vi "HIOKI PW3390 Conf Efficiency.vi"(0 "VISA Resource":refnum<visa-resource-name>, 1 "Set/Query (F: Set)":bool, 5 "Pin (0: P1)":T1(array[ring])=[enum."P1", enum."P1", enum."P1"], 7 "Pout (0: P1)":T1(array[ring])=[enum."P1", enum."P1", enum."P1"], 11 "error in (no error)":errorcluster, 12 "OPC query (T: ON)":bool=TRUE, 13 "Error Out (F: Off)":bool) -> (4 "VISA Resource out":refnum<visa-resource-name>, 6 "Pin out":T1(array[ring])=[enum."P1", enum."P1", enum."P1"], 8 "Pout out":T1(array[ring])=[enum."P1", enum."P1", enum."P1"], 15 "error out":errorcluster)   [LabVIEW 2009]
doc: "Sets and reads the Efficiency/Loss Calculation Formula. \n\nSet/Query\n Set: Send the setting commands for the device.\n Query: Query the setting of the device.\n\nPin\n Sets the Pin items of the Efficiency/Loss Calculation Formula for CH1 - CH3 in array.\n\nPout\n Sets the Pout items of the Efficiency/Loss Calculation Formula for CH1 - CH3 in array.\n\n<B>Note</B>\n P12/P34/P123 cannot be specified when they cannot be selected because of the wiring setting. Pm can only be specified during the implementation of the Motor Analysis Option and when Pm is selectable."
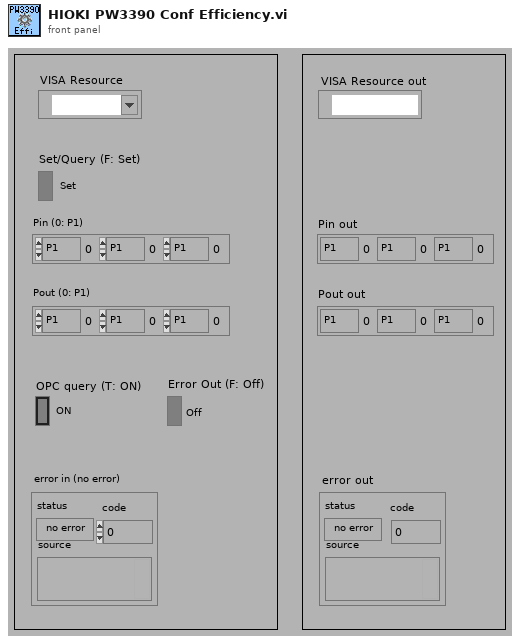
[diagram p1: front panel]
types:
  T1 = enum16{"P1", "P2", "P3", "P4", "P12", "P34", "P123", "Pm"}[]
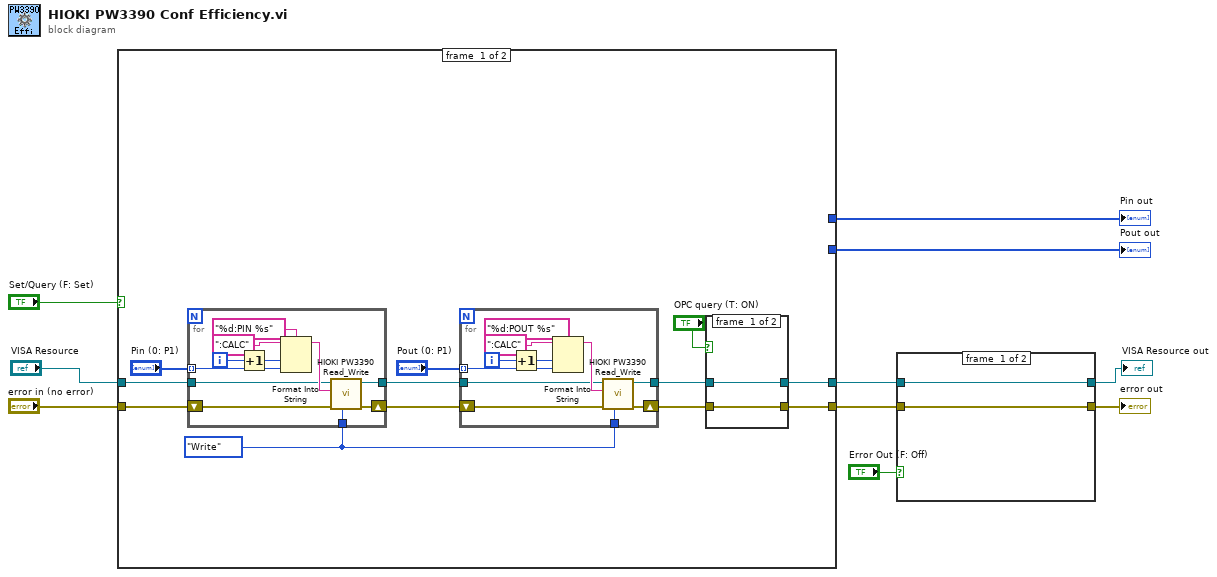
[diagram p0: block diagram]
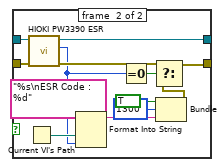
[diagram p2: hidden frame]
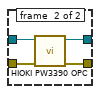
[diagram p3: hidden frame]
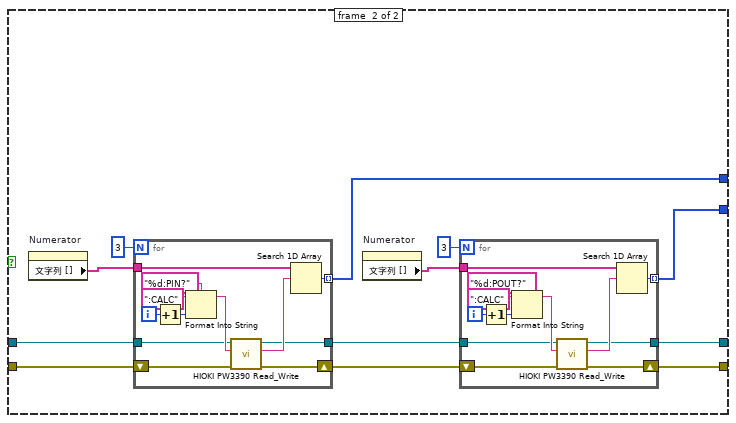
[diagram p4: hidden frame]
diagram:
  n1 = case shown="FALSE" "Set/Query (F: Set)" {
    tunnel: "error in (no error)" -> [w21 w60]
    tunnel: [w11 w53] -> w4
    tunnel: "VISA Resource" -> [w22 w61]
    tunnel: [w12 w57] -> w5
    tunnel: [_ w58] -> w8
    tunnel: [_ w54] -> w7
    frame #0 {
      w18 = enum16{"Read", "Write"}."Write" ("Read/Write")
      n2 = for {
        tunnel: "Pin (0: P1)" -> [w46] mode=indexing
        tunnel: w22 -> [w44]
        shift-right: [w43] -> w20
        shift-left: w21 -> [w42]
        tunnel: [w41] -> w19
        tunnel: w18 -> [w40]
        i -> [w48]
        n3 = Increment(x=w48) -> (x+1=w47:i32)
        n4 = Format Into String(format string="%d:PIN %s", initial string=":CALC", w47, w46) -> (resulting string=w45:string)  [unwired: 1 in, 1 out]
        n5 = call <instrlib>:"HIOKI PW3390 Read_Write.vi"("Read/Write"=w40, "error in (no error)"=w42, "data in"=w45, "VISA Resource"=w44) -> ("error out"=w43:errorcluster, "VISA Resource out"=w41:refnum<visa-resource-name>)  [unwired: 5 in, 1 out]
      }
      n6 = for {
        tunnel: "Pout (0: P1)" -> [w35] mode=indexing
        tunnel: w19 -> [w33]
        shift-right: [w32] -> w13
        shift-left: w20 -> [w31]
        tunnel: [w30] -> w14
        tunnel: w18 -> [w29]
        i -> [w37]
        n7 = Increment(x=w37) -> (x+1=w36:i32)
        n8 = Format Into String(format string="%d:POUT %s", initial string=":CALC", w36, w35) -> (resulting string=w34:string)  [unwired: 1 in, 1 out]
        n9 = call <instrlib>:"HIOKI PW3390 Read_Write.vi"("Read/Write"=w29, "error in (no error)"=w31, "data in"=w34, "VISA Resource"=w33) -> ("error out"=w32:errorcluster, "VISA Resource out"=w30:refnum<visa-resource-name>)  [unwired: 5 in, 1 out]
      }
      n10 = case shown="TRUE" "OPC query (T: ON)" {
        tunnel: [w24 w28] -> w12
        tunnel: [w23 w27] -> w11
        tunnel: w14 -> [w24 w26]
        tunnel: w13 -> [w23 w25]
        frame #0 {
        }
        frame #1 {
          n11 = call <instrlib>:"HIOKI PW3390 OPC.vi"("error in (no error)"=w25, "VISA Resource"=w26) -> ("error out"=w27:errorcluster, "VISA Resource out"=w28:refnum<visa-resource-name>)  [unwired: 7 in, 1 out]
        }
      }
    }
    frame #1 {
      # "Query"
      n12 = property on="Numerator" class="Enum (strict)"() -> ("文字列 []"=w62:string[])  [unwired: 2 in, 2 out]
      n13 = for {
        N: 3 -> [_]
        tunnel: [w86] -> w58 mode=indexing
        tunnel: w62 -> [w84]
        tunnel: w61 -> [w79]
        shift-right: [w77] -> w56
        shift-left: w60 -> [w78]
        tunnel: [w76] -> w59
        i -> [w81]
        n14 = Increment(x=w81) -> (x+1=w75:i32)
        n15 = Format Into String(format string="%d:PIN?", initial string=":CALC", w75) -> (resulting string=w80:string)  [unwired: 1 in, 1 out]
        n16 = call <instrlib>:"HIOKI PW3390 Read_Write.vi"("error in (no error)"=w78, "data in"=w80, "VISA Resource"=w79) -> ("error out"=w77:errorcluster, "data out"=w85:string, "VISA Resource out"=w76:refnum<visa-resource-name>)  [unwired: 6 in]
        n17 = Search 1D Array(1D array=w84, element=w85) -> (index of element=w86:i32)  [unwired: 1 in]
      }
      n18 = property on="Numerator" class="Enum (strict)"() -> ("文字列 []"=w55:string[])  [unwired: 2 in, 2 out]
      n19 = for {
        N: 3 -> [_]
        tunnel: [w74] -> w54 mode=indexing
        tunnel: w55 -> [w72]
        tunnel: w59 -> [w67]
        shift-right: [w65] -> w53
        shift-left: w56 -> [w66]
        tunnel: [w64] -> w57
        i -> [w69]
        n20 = Increment(x=w69) -> (x+1=w63:i32)
        n21 = Format Into String(format string="%d:POUT?", initial string=":CALC", w63) -> (resulting string=w68:string)  [unwired: 1 in, 1 out]
        n22 = call <instrlib>:"HIOKI PW3390 Read_Write.vi"("error in (no error)"=w66, "data in"=w68, "VISA Resource"=w67) -> ("error out"=w65:errorcluster, "data out"=w73:string, "VISA Resource out"=w64:refnum<visa-resource-name>)  [unwired: 6 in]
        n23 = Search 1D Array(1D array=w72, element=w73) -> (index of element=w74:i32)  [unwired: 1 in]
      }
    }
  }
  "Pin out" <- w8
  "Pout out" <- w7
  n24 = case shown="TRUE" "Error Out (F: Off)" {
    tunnel: w5 -> [w88 w101]
    tunnel: w4 -> [w87 w100]
    tunnel: [w87 w90] -> w3
    tunnel: [w88 w99] -> w1
    frame #0 {
    }
    frame #1 {
      n25 = Current VI's Path() -> (path=w97:path)
      n26 = call <instrlib>:"HIOKI PW3390 ESR.vi"("error in (no error)"=w100, "VISA Resource"=w101) -> ("error out"=w91:errorcluster, "Output Value"=w89:u8, "VISA Resource out"=w99:refnum<visa-resource-name>)  [unwired: 6 in, 1 out]
      n27 = Format Into String(format string="%s\nESR Code : %d", w97, w89) -> (resulting string=w93:string)  [unwired: 2 in, 1 out]
      n28 = Equal To 0?(x=w89) -> (x = 0?=w98:bool)
      n29 = Bundle("status"=TRUE, "code"=1300, w93) -> (w92:cluster{"status":bool, "code":i32, string})  [unwired: 1 in]
      n30 = Select(t=w91, s=w98, f=w92) -> (s? t:f=w90:errorcluster)
    }
  }
  "error out" <- w3
  "VISA Resource out" <- w1
